vi "h5_write_xwav_attributes.vi"(7 "object name":string, 8 "error in":errorcluster, 10 "xwave":T1={"attributes"=variant, "X"={"start"=0.0, "delta"=0.0, "units"="index", "dim"="au"}, "Y"={"data"=[], "units"="au"}}, 11 "h5 ref in":T2 format="%.0x") -> (0 "error out":errorcluster, 2 "dup xwave":T1={"attributes"=variant, "X"={"start"=0.0, "delta"=0.0, "units"="index", "dim"="au"}, "Y"={"data"=[], "units"="au"}}, 3 "dup h5 ref":T2 format="%.0x")   [LabVIEW 2015]
uses:
  <vilib>/addons/h5labview2/base/hid_t.ctl
  xwave/xwav.ctl
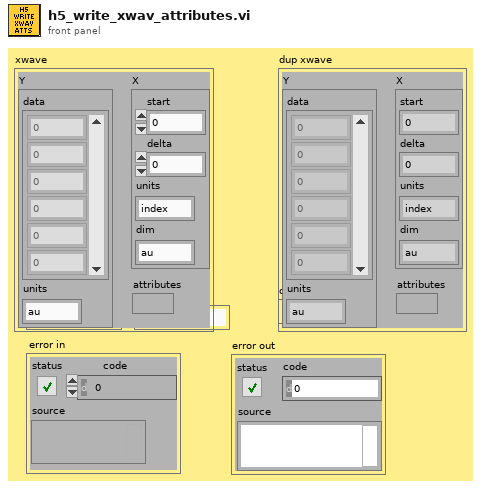
[diagram p1: front panel]
types:
  T1 = typedef "xwav.ctl" = cluster{"attributes":variant, "X":cluster{"start":dbl, "delta":dbl, "units":string, "dim":string}, "Y":cluster{"data":dbl[], "units":string}}
  T2 = typedef "hid_t.ctl" = i32
  T3 = cluster{"x0":dbl, "dx":dbl, "dimensions":string, "units":string}
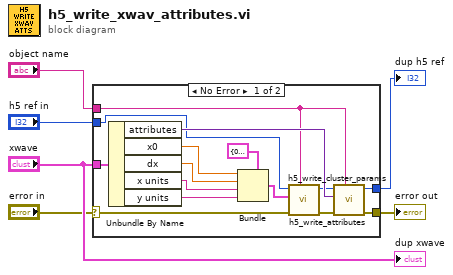
[diagram p0: block diagram]
diagram:
  n1 = case shown="No Error" "error in" {
    selector: "error in" -> [w8 w23]
    tunnel: [w11 w23] -> w6
    tunnel: "h5 ref in" -> [w9 w22]
    tunnel: "xwave" -> [w21 _]
    tunnel: "object name" -> [w10 _]
    tunnel: [w7 w22] -> w1
    frame No Error {
      n2 = Unbundle By Name(w21) -> ("attributes"=w14:variant, "x0"=w18:dbl, "dx"=w17:dbl, "x units"=w16:string, "y units"=w15:string)
      n3 = Bundle(cluster=T3 {"x0"=0.0, "dx"=0.0, "dimensions"="index", "units"="au"} ("xwave"), "x0"=w18, "dx"=w17, "dimensions"=w16, "units"=w15) -> (w19:T3)
      n4 = call "h5_write_cluster_params.vi"("object name"=w10, "error in (no error)"=w8, "cluster"=w19, "h5 ref"=w9) -> ("error out"=w13:errorcluster, "dup h5 ref"=w12:T2)  [unwired: 6 in]
      n5 = call "h5_write_attributes.vi"("object name"=w10, "error in"=w13, "attributes"=w14, "h5 ref"=w12) -> ("error out"=w11:errorcluster, "dup h5 ref"=w7:T2)  [unwired: 6 in]
    }
    frame Error {
    }
  }
  "dup h5 ref" <- w1
  "error out" <- w6
  "dup xwave" <- "xwave"
